vi "QCA - DUT Close NART.vi"(0 "CART TCP Connection":refnum<k5>, 11 "error in (no error)":errorcluster) -> (15 "error out":errorcluster)   [LabVIEW 2012]
uses:
  NART Constants.vi
panel:
  out "standard error":string
  out "standard output":string
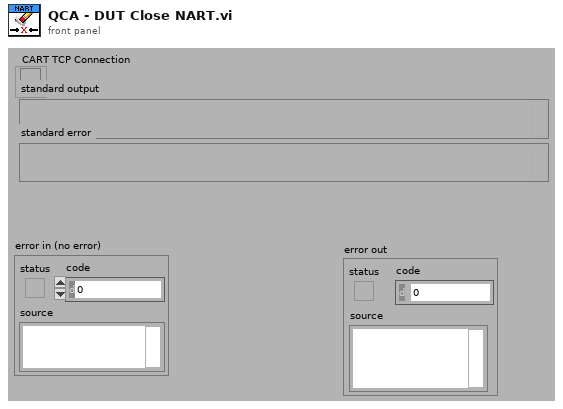
[diagram p1: front panel]
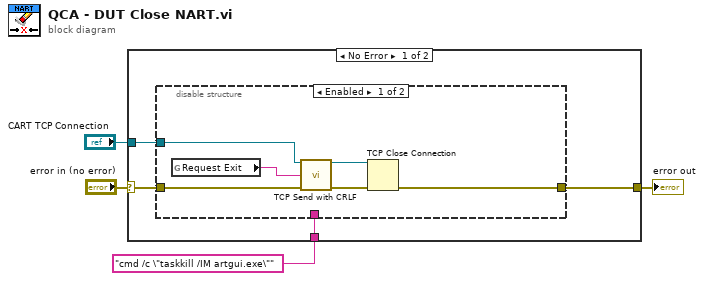
[diagram p0: block diagram]
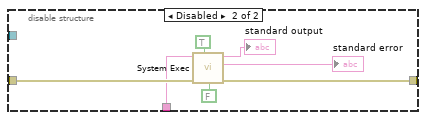
[diagram p2: hidden frame]
diagram:
  n1 = case shown="No Error" "error in (no error)" {
    selector: "error in (no error)" -> [w8 w22]
    tunnel: [w7 w22] -> w3
    tunnel: "CART TCP Connection" -> [w6 _]
    tunnel: "cmd /c \"taskkill /IM artgui.exe\"" ("format string") -> [w5 _]
    frame No Error {
      n2 = disable-structure shown="Enabled" {
        disable-tunnel: w8 -> [w14 w21]
        disable-tunnel: [w12 w15] -> w7
        disable-tunnel: w6 -> [w10 _]
        disable-tunnel: w5 -> [_ w19]
        frame Enabled {
          n3 = global read "NART Constants.vi" "Request Exit"() -> (w9:string)
          n4 = call "TCP Send with CRLF.vi"("CART TCP Connection"=w10, "data in"=w9, "error IO"=w14) -> ("CART TCP Connection Out"=w11:refnum<k5>, "error out"=w13:errorcluster)  [unwired: 11 in]
          n5 = TCP Close Connection(connection ID=w11, error in (no error)=w13) -> (error out=w12:errorcluster)  [unwired: 1 in, 1 out]
        }
        frame Disabled {
          n6 = call <vilib>:"System Exec.vi"("run minimized? (F)"=FALSE, "wait until completion? (T)"=TRUE, "error in (no error)"=w21, "command line"=w19) -> ("error out"=w15:errorcluster, "standard error"=→"standard error":string, "standard output"=→"standard output":string)  [unwired: 4 in, 1 out]
        }
      }
    }
    frame Error {
    }
  }
  "error out" <- w3
